vi "thermistor transfer function.vi"(0 "B":fxp<+/-,32,16>, 5 "1/R_inf":fxp<+,32,7>, 7 "V":fxp<+/-,24,5>, 9 "input valid":bool=TRUE, 11 "ready for output (T)":bool=TRUE) -> (8 "Temperature":fxp<+/-,32,16>, 10 "output valid":bool, 15 "ready for input":bool)   [LabVIEW 2018]
uses:
  <vilib>/rvi/FXPMathLib/FxpDiv/subVIs/nifxpmath_Div_SimConfig.ctl
  <vilib>/rvi/FXPMathLib/FxpDiv/simVIs/DllFxpDivTemp_sub.vi
  <vilib>/rvi/FXPMathLib/FxpDiv/XNode/nifxpmath_Div.xnode
  <vilib>/rvi/FXPMathLib/FxpSub/XNode/nifxpmath_Sub.xnode
  <vilib>/rvi/FXPMathLib/sim/FxpSim.dll
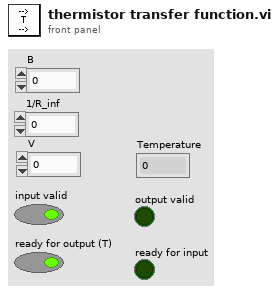
[diagram p1: front panel]
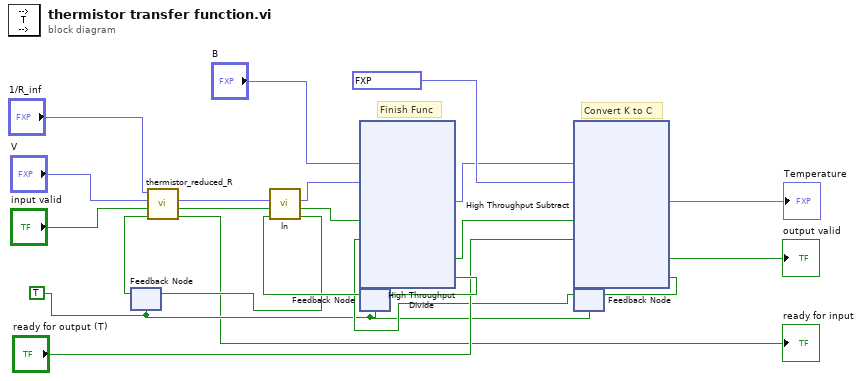
[diagram p0: block diagram]
diagram:
  w10 = TRUE
  # "Finish Func"
  # "Convert K to C"
  n1 = feedback #1(w10) -> (w9:bool)
  n2 = call "thermistor_reduced_R.vi"("ready for output (T)"=w9, "input valid"="input valid", "V"="V", "1/R_inf"="1/R_inf") -> ("ready for input"=→"ready for input":bool, "output valid"=w4:bool, "R^~"=w3:fxp<+/-,64,32>)  [unwired: 5 in]
  n3 = feedback #2(w10) -> (w21:bool)
  n4 = call "ln.vi"("ready for output (T)"=w21, "input valid"=w4, "x"=w3) -> ("ready for input"=w20:bool, "output valid"=w1:bool, "ln(x)"=w2:fxp<+/-,32,16>)  [unwired: 6 in]
  n5 = feedback-in #1(w20) -> ()
  n6 = feedback #3(w10) -> (w11:bool)
  n7 = xnode "High Throughput Divide"("x"="B", "y"=w2, "input valid"=w1, "ready for output (T)"=w11) -> ("x/y"=w16:fxp<+/-,32,16>, "output valid"=w15:bool, "ready for input"=w22:bool)
  n8 = feedback-in #2(w22) -> ()
  n9 = xnode "High Throughput Subtract"("x"=w16, "y"=fxp<+,16,9> 273.1484375, "input valid"=w15, "ready for output (T)"="ready for output (T)") -> ("x-y"=→"Temperature":fxp<+/-,32,16>, "output valid"=→"output valid":bool, "ready for input"=w12:bool)
  n10 = feedback-in #3(w12) -> ()
